vi "WFComposeA.vi"(8 "error in (no error)":errorcluster, 10 "WFRepetitions":T1={"Del (s)"=0.0, "Int (s)"=0.0, "N"=1} {"Int (s)" min=0.0 format="%#_4g"; "Del (s)" min=0.0 format="%#_4f"}, 11 "Waveform In":waveform(dbl)={"t0"=timestamp(0 s since 1904-01-01), "dt"=0.0, "Y"=[]}) -> (0 "error out":errorcluster, 3 "Analog Waveform Out":waveform(dbl))   [LabVIEW 2013]
uses:
  WFRepetitions.ctl
  WFComposeCanA.vi
  WFGetDtFsA.vi
  <vilib>/Waveform/WDTOps.llb/WDT Waveform Duration DBL.vi
  <vilib>/Waveform/WDTOps.llb/WDT Number of Waveform Samples DBL.vi
  WFAppend2A.vi
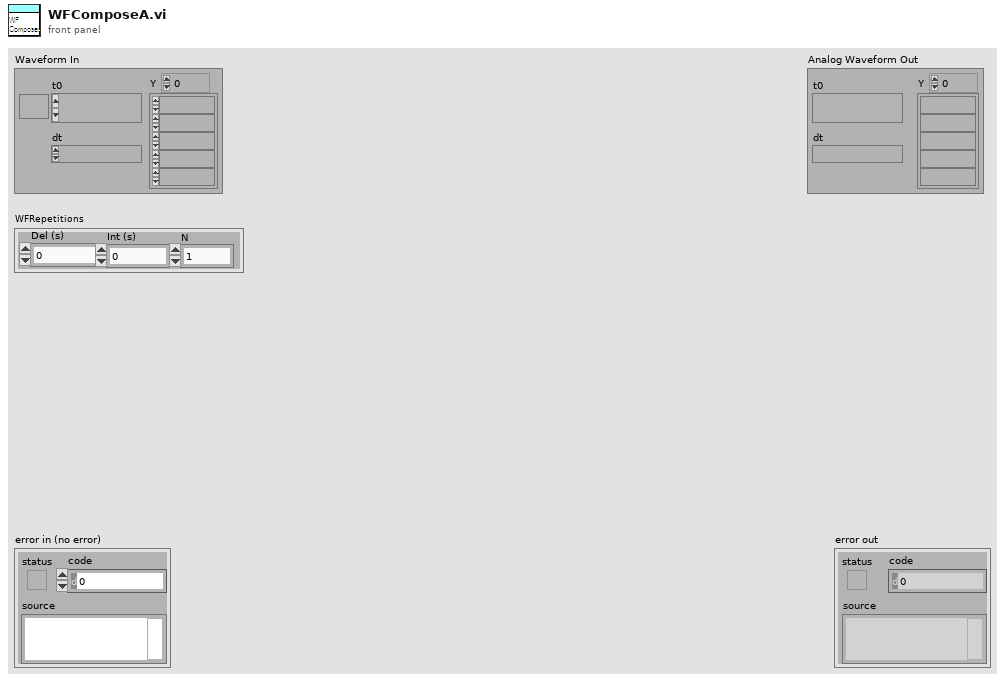
[diagram p1: front panel]
types:
  T1 = typedef "WFRepetitions.ctl" = cluster{"Del (s)":dbl, "Int (s)":dbl, "N":i32}
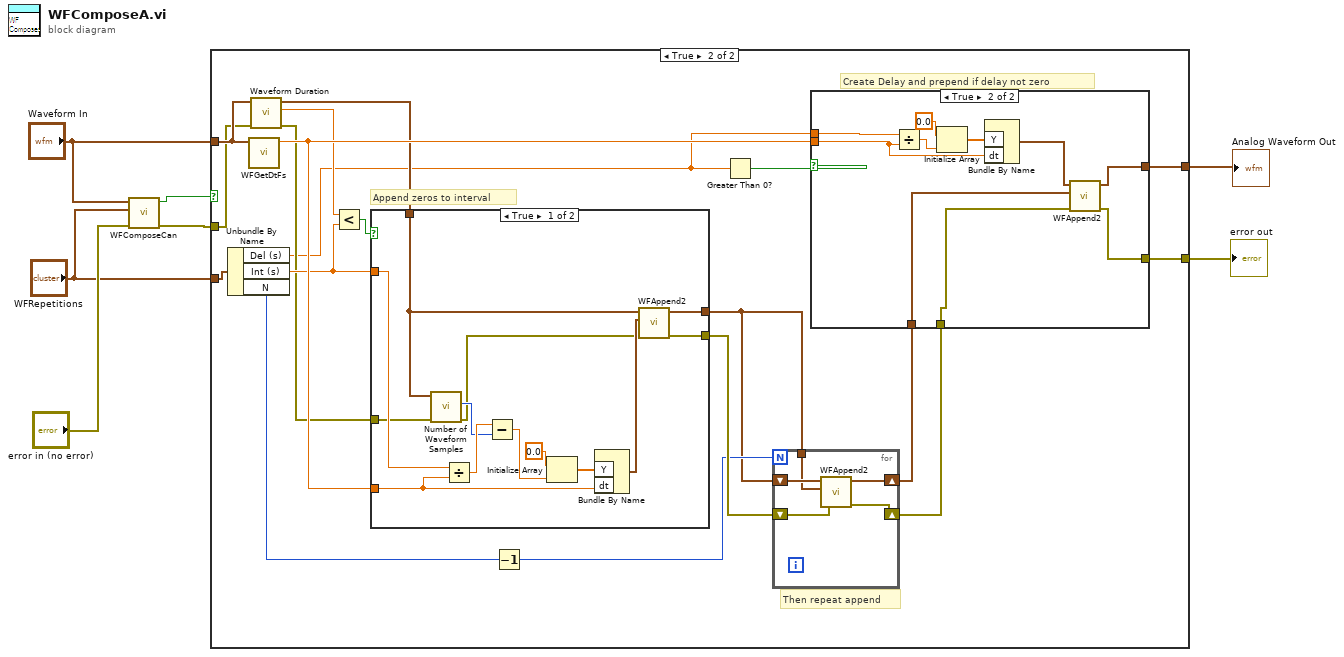
[diagram p0: block diagram]
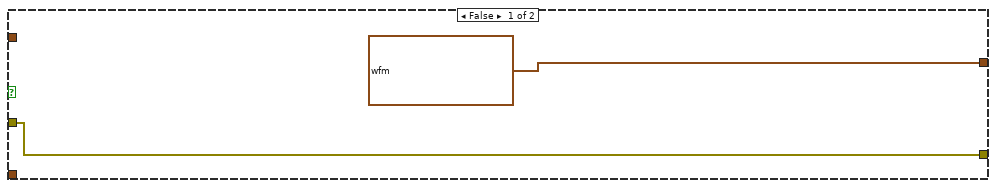
[diagram p2: hidden frame]
diagram:
  n1 = call-poly "WFComposeCan.vi"("error in (no error)"="error in (no error)", "Cluster"="WFRepetitions", "Waveform In"="Waveform In") -> ("error out"=w4:errorcluster, "ComposeCan"=w6:bool)  [unwired: 7 in]
  n2 = case shown="True" w6 {
    tunnel: [waveform(dbl) {"t0"=timestamp(0 s since 1904-01-01), "dt"=1.0, "Y"=[]} ("Waveform") w13] -> w7
    tunnel: w4 -> [w8 w19]
    tunnel: [w8 w11] -> w3
    tunnel: "Waveform In" -> [_ w24]
    tunnel: "WFRepetitions" -> [_ w25]
    frame False {
    }
    frame True {
      # "Then repeat append"
      # "Create Delay and prepend if delay not zero"
      # "Append zeros to interval"
      n3 = Unbundle By Name(w25) -> ("Del (s)"=w10:dbl, "Int (s)"=w20:dbl, "N"=w17:i32)
      n4 = call-poly "WFGetDtFs.vi"("Waveform"=w24) -> ("dt"=w27:dbl)  [unwired: 9 in, 1 out]
      n5 = call-poly <vilib>:"Waveform Duration.vi"("error in (no error)"=w19, "waveform in"=w24) -> ("error out"=w18:errorcluster, "duration"=w23:dbl, "waveform out"=w21:waveform(dbl))  [unwired: 7 in]
      n6 = Less?(x=w23, y=w20) -> (x < y?=w22:bool)
      n7 = case shown="True" w22 {
        tunnel: w27 -> [w44 _]
        tunnel: [w39 w47] -> w26
        tunnel: [w38 w48] -> w15
        tunnel: w21 -> [w36 w48]
        tunnel: w20 -> [w37 _]
        tunnel: w18 -> [w35 w47]
        frame True {
          n8 = call-poly <vilib>:"Number of Waveform Samples.vi"("error in (no error)"=w35, "waveform in"=w36) -> ("error out"=w34:errorcluster, "number of samples"=w42:i32)  [unwired: 7 in, 1 out]
          n9 = Divide(x=w37, y=w44) -> (x/y=w43:dbl)
          n10 = Subtract(x=w43, y=w42) -> (x-y=w41:dbl)
          n11 = Initialize Array(0.0 ("element"), w41) -> (w46:dbl[])
          n12 = Bundle By Name("Y"=w46, "dt"=w44) -> (w40:waveform(dbl))  [unwired: 1 in]
          n13 = call-poly "WFAppend2.vi"("error in (no error)"=w34, "Waveform In 2"=w40, "Waveform In"=w36) -> ("error out"=w39:errorcluster, "Waveform Out"=w38:waveform(dbl))  [unwired: 3 in]
        }
        frame False {
        }
      }
      n14 = Decrement(x=w17) -> (x-1=w16:i32)
      n15 = Greater Than 0?(x=w10) -> (x > 0?=w28:bool)
      n16 = for {
        N: w16 -> [_]
        shift-right: [w32] -> w14
        shift-left: w15 -> [w33]
        shift-right: [w30] -> w12
        shift-left: w26 -> [w31]
        tunnel: w15 -> [w29]
        n17 = call-poly "WFAppend2.vi"("error in (no error)"=w31, "Waveform In 2"=w29, "Waveform In"=w33) -> ("error out"=w30:errorcluster, "Waveform Out"=w32:waveform(dbl))  [unwired: 3 in]
      }
      n18 = case shown="True" w28 {
        tunnel: w27 -> [_ w57]
        tunnel: w14 -> [w50 w55]
        tunnel: [w50 w54] -> w13
        tunnel: w12 -> [w49 w53]
        tunnel: [w49 w52] -> w11
        tunnel: w10 -> [_ w51]
        frame False {
        }
        frame True {
          n19 = Divide(x=w51, y=w57) -> (x/y=w58:dbl)
          n20 = Initialize Array(0.0 ("element"), w58) -> (w60:dbl[])
          n21 = Bundle By Name("Y"=w60, "dt"=w57) -> (w56:waveform(dbl))  [unwired: 1 in]
          n22 = call-poly "WFAppend2.vi"("error in (no error)"=w53, "Waveform In 2"=w55, "Waveform In"=w56) -> ("error out"=w52:errorcluster, "Waveform Out"=w54:waveform(dbl))  [unwired: 3 in]
        }
      }
    }
  }
  "error out" <- w3
  "Analog Waveform Out" <- w7
